vi "Write Device Identification.vi"(8 "error in (no error)":errorcluster, 10 "objects":cluster{"object ID":u8, "value":string}[](array[cluster]) {"object ID" format="%x"}, 11 "Modbus slave in":refnum<class "Modbus Slave.lvclass">) -> (0 "error out":errorcluster, 3 "Modbus slave out":refnum<class "Modbus Slave.lvclass">)   [LabVIEW 2020, in "Modbus Slave.lvclass"]
doc: "Writes the device identification of a Modbus slave. Device identification consists of data elements called objects. Each object has an identification number and stores Modbus slave information."
uses:
  <vilib>/Modbus/slave/Modbus Slave.lvclass
  <vilib>/Modbus/slave/Modbus Slave.lvclass/Modbus Slave.ctl
  <vilib>/Modbus/subvis/Data and Functions/Device Data Model/Device Data Model.lvclass
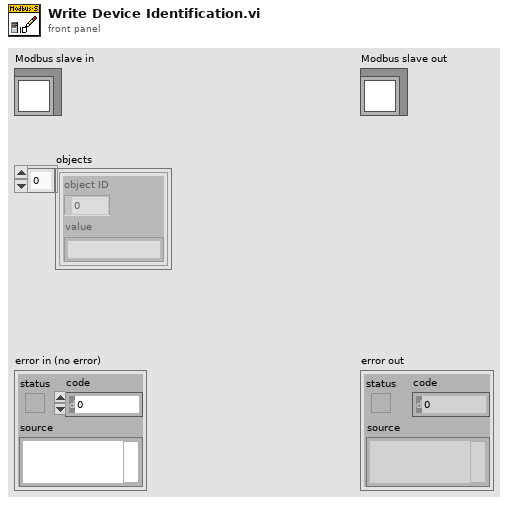
[diagram p1: front panel]
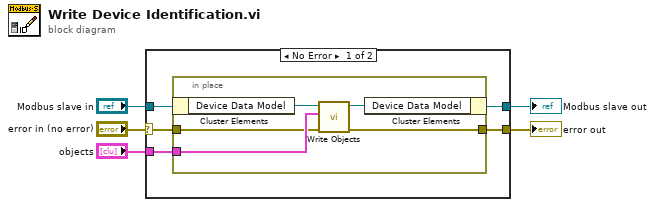
[diagram p0: block diagram]
diagram:
  n1 = case shown="No Error" "error in (no error)" {
    selector: "error in (no error)" -> [w6 w17]
    tunnel: [w10 w16] -> w5
    tunnel: "Modbus slave in" -> [w9 w16]
    tunnel: [w8 w17] -> w3
    tunnel: "objects" -> [w7 _]
    frame No Error {
      n2 = in-place {
        in-place-border: [w15] -> w8
        in-place-border: w7 -> [w14]
        in-place-border: w6 -> [w12]
        n3 = in-place-cluster #1(w9) -> ("Device Data Model"=w13:refnum<class "Device Data Model.lvclass">)
        n4 = call-dynamic "Write Objects.vi"("error in (no error)"=w12, "objects"=w14, "device data model in"=w13) -> ("error out"=w15:errorcluster, "device data model out"=w11:refnum<class "Device Data Model.lvclass">)  [unwired: 7 in]
        n5 = in-place-cluster #1("Device Data Model"=w11) -> (w10:refnum<class "Modbus Slave.lvclass">)
      }
    }
    frame Error {
    }
  }
  "error out" <- w3
  "Modbus slave out" <- w5
